vi "Step2_3_BandPass_AntiHarmonic.vi"(9 "s_axis_data_tdata":fxp<+/-,40,2>, 10 "s_axis_data_tvalid":bool) -> (1 "m_axis_data_tdata":fxp<+/-,24,3>, 2 "m_axis_data_tvalid":bool, 3 "s_axis_data_tready":bool)   [LabVIEW 2018]
uses:
  <vilib>/rvi/XilinxIP/XIPIN_XNode/niFpgaXIPIN.xnode
  Deprecated_Delete/DigitalFilterDesign/FIR_Filter_Configuration/FIR Compiler/xsim.dir/FIR_Compiler_3CE652926F5B43F18022D1349C670FA0/xsimk_3CE652926F5B43F18022D1349C670FA0.dll
  <vilib>/rvi/IPIntegrationNode/IPINode_Xnode/niFpgaIPINode.xnode
  <vilib>/rvi/IPIntegrationNode/IPINode_Typedef/niFpgaIPINodeSupportedFamilies.ctl
  <vilib>/rvi/IPIntegrationNode/IPINode_Utilities/niFpgaIPINodeSimCore.vi
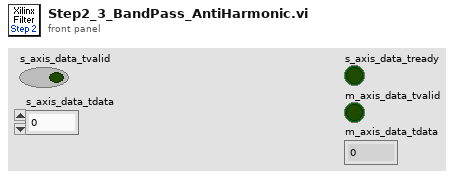
[diagram p1: front panel]
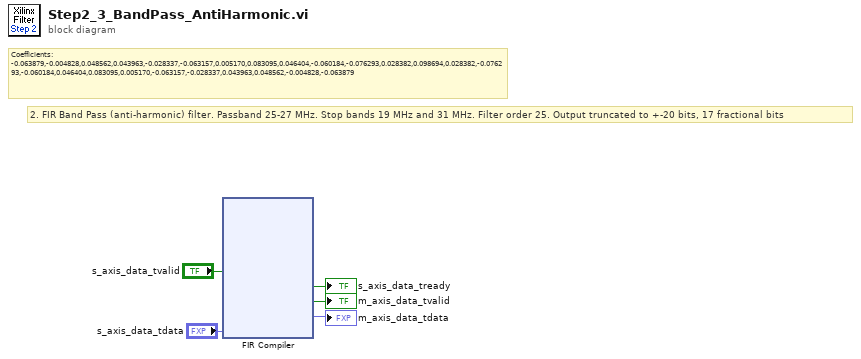
[diagram p0: block diagram]
diagram:
  # "2.\tFIR Band Pass (anti-harmonic) filter. Passband 25-27 MHz. Stop bands 19 MHz and 31 MHz. Filter order 25. Output truncated to +-20 bits, 17 fractional bits"
  # "Coefficients: -0.063879,-0.004828,0.048562,0.043963,-0.028337,-0.063157,0.005170,0.083095,0.046404,-0.060184,-0.076293,0.028382,0.098694,0.028382,-0.076293,-0.060184,0.046404,0.083095,0.005170,-0.063157,-0.028337,0.043963,0.048562,-0.004828,-0.063879"
  n1 = xnode ("FIR Compiler")("s_axis_data_tvalid"="s_axis_data_tvalid", "s_axis_data_tdata"="s_axis_data_tdata") -> ("s_axis_data_tready"=→"s_axis_data_tready":bool, "m_axis_data_tvalid"=→"m_axis_data_tvalid":bool, "m_axis_data_tdata"=→"m_axis_data_tdata":fxp<+/-,24,3>)
